vi "Read 2nd image mirror axis.vi"(8 "error in (no error)":errorcluster, 11 "Correct params in":refnum<class "CV-Correction.lvclass">) -> (0 "error out":errorcluster, 2 "2nd image mirror axis":u32(ring)=1 items=["Horizontal", "Vertical", "Central", "1st Diagonal", "2nd Diagonal"], 3 "Correct params out":refnum<class "CV-Correction.lvclass">)   [LabVIEW 2013, in "CameraVision.lvlib" / "CV-Correction.lvclass"]
uses:
  CV-Correction.lvclass
  CV-Correction.lvclass/CV-Correction.ctl
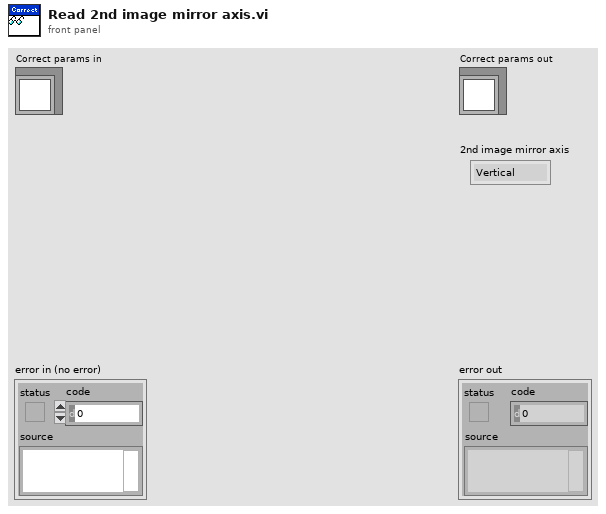
[diagram p1: front panel]
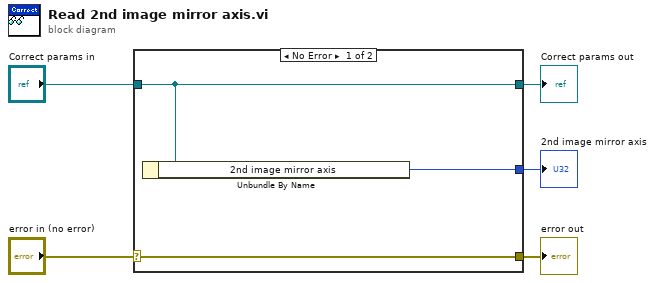
[diagram p0: block diagram]
diagram:
  n1 = case shown="No Error" "error in (no error)" {
    selector: "error in (no error)" -> [w8 w9]
    tunnel: [w8 w9] -> w4
    tunnel: [w7 w10] -> w2
    tunnel: "Correct params in" -> [w7 w10]
    tunnel: [w6 _] -> w1
    frame No Error {
      n2 = Unbundle By Name(w7) -> ("2nd image mirror axis"=w6:u32)
    }
    frame Error {
    }
  }
  "error out" <- w4
  "Correct params out" <- w2
  "2nd image mirror axis" <- w1
